vi "set subNodes.vi"(8 "error in (no error)":errorcluster, 10 "subNodes[]*":refnum<data-value>[](array[refnum]), 11 "xceNode in":refnum<class "xceNode.lvclass">) -> (0 "error out":errorcluster, 3 "xceNode out":refnum<class "xceNode.lvclass">)   [LabVIEW 2013, in "xceNode.lvclass"]
doc: "Sets subNode. subNodeare data value references to xceNodes that resides below this node in the tree data structure."
uses:
  xceNode.lvclass
  xceTreeObj/xceTreeObj.lvclass
  xceNode.lvclass/xceNode.ctl
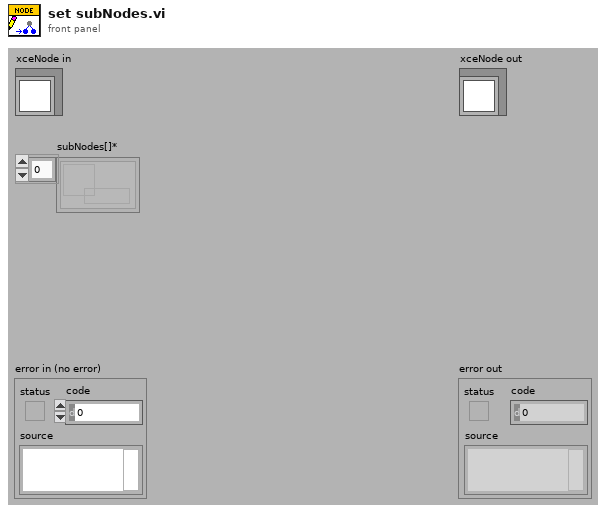
[diagram p1: front panel]
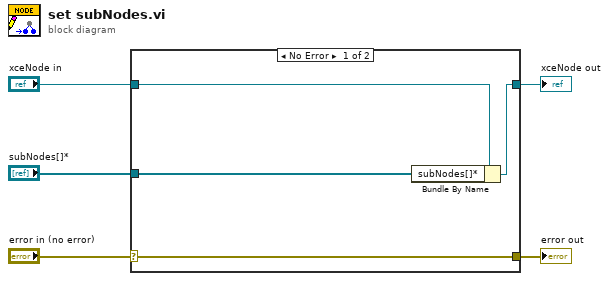
[diagram p0: block diagram]
diagram:
  n1 = case shown="No Error" "error in (no error)" {
    selector: "error in (no error)" -> [w9 w10]
    tunnel: [w9 w10] -> w4
    tunnel: [w7 w11] -> w2
    tunnel: "xceNode in" -> [w8 w11]
    tunnel: "subNodes[]*" -> [w6 _]
    frame No Error {
      n2 = Bundle By Name(cluster=w8, "subNodes[]*"=w6) -> (w7:refnum<class "xceNode.lvclass">)
    }
    frame Error {
    }
  }
  "error out" <- w4
  "xceNode out" <- w2
